vi "Configure Serial Bus (SPI - Basic).vi"(0 "VISA resource name":refnum<visa-resource-name>, 1 "Framing Type (0: Chip Select)":i32(ring) items=["Chip Select", "Not Chip Select", "Timeout"], 2 "Data Length (8 Bytes)":dbl=8.0, 5 "Serial Bus Name (1: Serial Bus 1)":i32(ring)=1 items=["Serial Bus 1"=1, "Serial Bus 2"=2], 7 "Bit Order (0: LSB First)":i32(ring) items=["LSB First", "MSB First"], 9 "Clock Edge (0: Positive)":i32(ring) items=["Positive", "Negative"], 11 "error in (no error)":errorcluster, 12 "Timeout (1E-5 S)":dbl=1e-05) -> (4 "VISA resource name out":refnum<visa-resource-name>, 15 "error out":errorcluster)   [LabVIEW 2017, in "Agilent 2000 3000 X-Series.lvlib"]
doc: "Configures the basic settings of SPI bus."
uses:
  Agilent 2000 3000 X-Series.lvlib
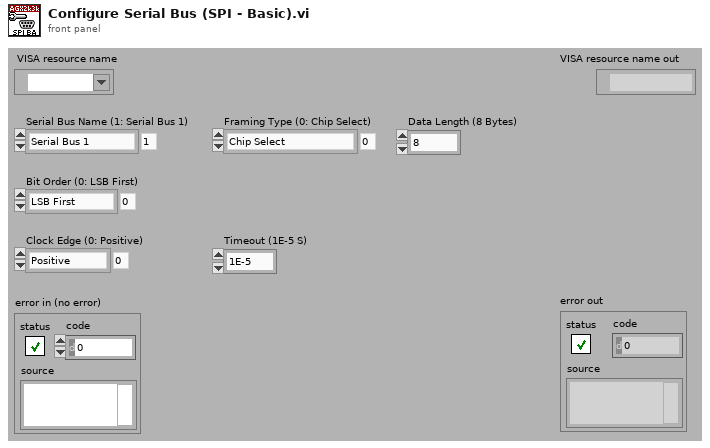
[diagram p1: front panel]
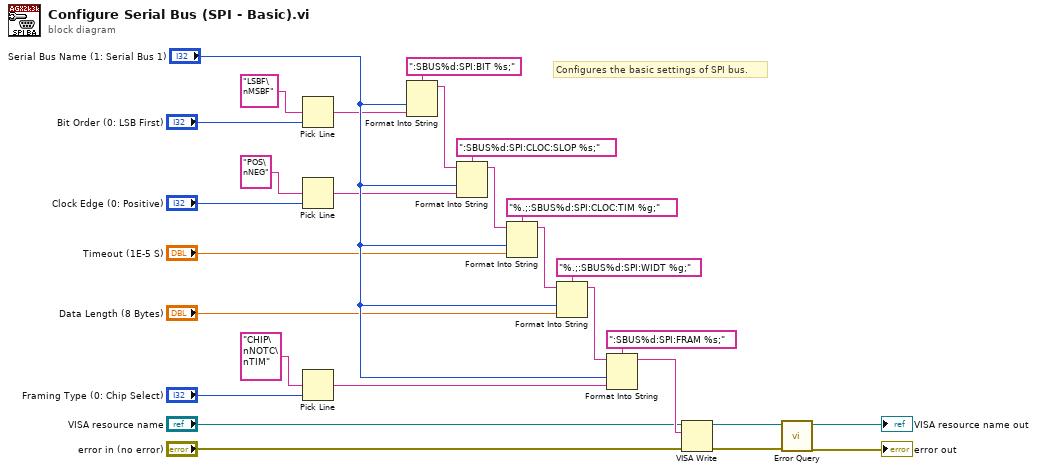
[diagram p0: block diagram]
diagram:
  # "Configures the basic settings of SPI bus."
  n1 = Pick Line(multi-line string="LSBF\nMSBF", line index="Bit Order (0: LSB First)") -> (output string=w24:string)  [unwired: 1 out]
  n2 = Pick Line(multi-line string="POS\nNEG", line index="Clock Edge (0: Positive)") -> (output string=w19:string)  [unwired: 1 out]
  n3 = Pick Line(multi-line string="CHIP\nNOTC\nTIM", line index="Framing Type (0: Chip Select)") -> (output string=w8:string)  [unwired: 1 out]
  n4 = Format Into String(format string=":SBUS%d:SPI:BIT %s;", "Serial Bus Name (1: Serial Bus 1)", w24) -> (resulting string=w21:string)  [unwired: 2 in, 1 out]
  n5 = Format Into String(format string=":SBUS%d:SPI:CLOC:SLOP %s;", initial string=w21, "Serial Bus Name (1: Serial Bus 1)", w19) -> (resulting string=w18:string)  [unwired: 1 in, 1 out]
  n6 = Format Into String(format string="%.;:SBUS%d:SPI:CLOC:TIM %g;", initial string=w18, "Serial Bus Name (1: Serial Bus 1)", "Timeout (1E-5 S)") -> (resulting string=w15:string)  [unwired: 1 in, 1 out]
  n7 = Format Into String(format string="%.;:SBUS%d:SPI:WIDT %g;", initial string=w15, "Serial Bus Name (1: Serial Bus 1)", "Data Length (8 Bytes)") -> (resulting string=w10:string)  [unwired: 1 in, 1 out]
  n8 = Format Into String(format string=":SBUS%d:SPI:FRAM %s;", initial string=w10, "Serial Bus Name (1: Serial Bus 1)", w8) -> (resulting string=w7:string)  [unwired: 1 in, 1 out]
  n9 = VISA Write(VISA resource name="VISA resource name", write buffer=w7, error in (no error)="error in (no error)") -> (VISA resource name out=w4:refnum<visa-resource-name>, error out=w3:errorcluster)  [unwired: 1 out]
  n10 = call "Error Query.vi"("error in (no error)"=w3, "VISA resource name"=w4) -> ("error out"=→"error out":errorcluster, "VISA resource name out"=→"VISA resource name out":refnum<visa-resource-name>)  [unwired: 8 out]
